vi "Package Version.vi"() -> (2 "Package Version":string="0.1.0")   [LabVIEW 2020]
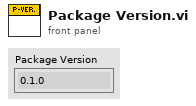
[diagram p1: front panel]
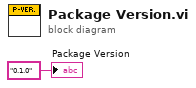
[diagram p0: block diagram]
diagram:
  "Package Version" <- "0.1.0" ("Current Package Version")
